vi "VI Server_Test_Slots_TREE_PopulateTreeItems.vi"(4 "Item Names":string[][](array[string])=[["Setting NI-USB6343 digital and analog outputs", "0", "", "", "", "", "", ""], ["Setting digital output and input", "1", "Sets port 0/line 1 to Hi", "Digital input port0/line0 shall be Hi", "", "", "", ""], ["DPO2012B,SET,OS.Ch2.Enbl,ON,", "1", "NI-USB6343,SET,AO.SampleMode,Continious Samples,", "NI-USB6343,SET,AO.MaxVoltage,10.000,", "", "", "", ""], ["DPO2012B: Get the waveform for Graph 2", "1", "Gets the waveform for Graph 2 from DPO2012B.", "", "", "", "", ""], ["Keithley2100,SET,*RST,ON,", "1", "NI-USB6343,SET,AO.Output,OFF,", "NI-USB6343,SET,AO.Physical.Channel,NI-USB6343/ao1,", "", "", "", ""], ["Test EXI-8000PCI MIL-1553 Board", "0", "EXI-8000PCI MIL-1553 Board module 0 shall be set as BC (Buss Controller) and the module 1 shall be set as RT.", "The board shall perform BC2RT, RT2BC and BM (bus monitor) functions.", "", "", "", ""], ["EXI-8000PCIe,SET,RT.Start,OFF,", "2", "EXI-8000PCIe,SET,BC.Mode,BC/CONCURRENT RT,", "EXI-8000PCIe,SET,BC.RT.Number,1,", "", "", "", ""], ["EXI-8000PCIe,SET,RT.Start,OFF,", "2", "EXI-8000PCIe,SET,BC.Mode,BC/CONCURRENT RT,", "EXI-8000PCIe,SET,BC.RT.Number,1,", "", "", "", ""], ["Delay,,,250,", "1", "EXI-8000PCIe,SET,BC.Mode,BC/CONCURRENT RT,", "EXI-8000PCIe,SET,BC.RT.Number,1,", "", "", "", ""], ["EXI-8000PCIe,SET,RT.Start,OFF,", "1", "EXI-8000PCIe,SET,BC.Mode,BC/CONCURRENT RT,", "EXI-8000PCIe,SET,BC.RT.Number,1,", "", "", "", ""], ["Test SRS 5330A and API 8810A", "0", "Testing synchroresolver instruments", "", "", "", "", ""], ["Setting SRS 5330A", "1", "Testing SRS 5330A functions", "Testing SRS 5330A functions", "", "", "", ""], ["API 8810A Functions test", "1", "Perfoms API 8810A Functions test", "", "", "", "", ""], ["Demo test", "1", "Demo Test: create test case", "", "", "", "", ""], ["DPO2012B,SET,OS.Ch2.Enbl,ON,", "1", "NI-USB6343,SET,AO.SampleMode,Continious Samples,", "NI-USB6343,SET,AO.MaxVoltage,10.000,", "", "", "", ""]], 6 "Tree.RowHeaders":string[](array[string]), 7 "Label":string="Test.Tree", 8 "error in":errorcluster, 9 "Tree.Ref":refnum<vi>, 11 "VI Server.RefsCluster":T1={"Labels"=["Tab.Main", "EXIT", "Test.Start", "Test.ABORT", "Test.Pause", "error in", "error out", "Login.Level", "Login.Name", "TestConfiguration.TestCaseEdit", "TestConfiguration.DeleteTestCase", "TestConfiguration.P/N.TestCaseNew", "TestConfiguration.SaveTestCase", "Settings.TestCase.Refresh", "Help", "System.Message", "Instruments.Status", "Test.Tree", "Serial#", "Test.P/N", "Messages & Status", "Settings.P/N", "TestCase", "TestConfiguration", "TestCase.Description", "TestCase.Conditions", "TestCase.Parameter", "TestCaseConfiguration", "TestCase.TraceLimits", "TestCase.Function", "TestCase.Function.Argument1", "TestCase.Function.Argument2", "TestCase.Function.Argument3", "TestCase.Function.Argument3.DBL", "TestCase.LimitsIndex", "LimitsIndex.New", "Limit.Hi", "Limit.Lo", "Limit.Units", "Limits.SAVE", "Limits.Remove", "TestCase.Instrument.Data", "TestCase.InstrumentData.InRange", "TestCase.Execute.Selected", "TestCase.Execute.All", "TestCase.Execute.Pause", "TestCase.Execute.ABORT", "TestCase.Execute.Instruction", "TestCase.Add.Instruction", "TestCase.SAVE", "TestCase.Instrument.Data.Array", "TestCase.Execution.StepTime", "TestCase.Update.Instruction", "Limit.Message", "TestCase.Execute.Pass/Fail", "Performance.Verification.Pass/Fail", "Performance.Verification.SAVE", "TestCase.Execute.Next", "TestConfiguration.RunAll", "TestConfiguration.Execute.Pass/Fail", "TestCaseExecution.StopOnFailure", "TestConfiguration.Run.Step", "TestCase.Add.Instruction.Pos", "TestCase.Execute.Steps", "TestCase.Execute.Step.Pause", "Graph1", "Graph2", "Image1", "Image2", "Image3", "Mem1", "Mem2", "Mem3", "Mem4", "Mem5", "Mem6", "Mem7", "Mem8", "Mem9", "Mem10", "Mem11", "Mem12", "Mem13", "Mem14", "Mem15", "Mem16", "Mem97", "Mem98", "Mem99", "Mem100", "Mem101", "Mem102", "Mem103", "Mem104", "Mem105", "Mem106", "Mem107", "Mem108", "Mem109", "Mem110", "Mem111", "Mem112", "Mem17", "Mem18", "Mem19", "Mem20", "Mem21", "Mem22", "Mem23", "Mem24", "Mem25", "Mem26", "Mem27", "Mem28", "Mem29", "Mem30", "Mem31", "Mem32", "Mem113", "Mem114", "Mem115", "Mem116", "Mem117", "Mem118", "Mem119", "Mem120", "Mem121", "Mem122", "Mem123", "Mem124", "Mem125", "Mem126", "Mem127", "Mem128", "Mem33", "Mem34", "Mem35", "Mem36", "Mem37", "Mem38", "Mem39", "Mem40", "Mem41", "Mem42", "Mem43", "Mem44", "Mem45", "Mem46", "Mem47", "Mem48", "Mem129", "Mem130", "Mem131", "Mem132", "Mem133", "Mem134", "Mem135", "Mem136", "Mem137", "Mem138", "Mem139", "Mem140", "Mem141", "Mem142", "Mem143", "Mem144", "Mem49", "Mem50", "Mem51", "Mem52", "Mem53", "Mem54", "Mem55", "Mem56", "Mem57", "Mem58", "Mem59", "Mem60", "Mem61", "Mem62", "Mem63", "Mem64", "Mem145", "Mem146", "Mem147", "Mem148", "Mem149", "Mem150", "Mem151", "Mem152", "Mem153", "Mem154", "Mem155", "Mem156", "Mem157", "Mem158", "Mem159", "Mem160", "Mem65", "Mem66", "Mem67", "Mem68", "Mem69", "Mem70", "Mem71", "Mem72", "Mem73", "Mem74", "Mem75", "Mem76", "Mem77", "Mem78", "Mem79", "Mem80", "Mem161", "Mem162", "Mem163", "Mem164", "Mem165", "Mem166", "Mem167", "Mem168", "Mem169", "Mem170", "Mem171", "Mem172", "Mem173", "Mem174", "Mem175", "Mem176", "Mem81", "Mem82", "Mem83", "Mem84", "Mem85", "Mem86", "Mem87", "Mem88", "Mem89", "Mem90", "Mem91", "Mem92", "Mem93", "Mem94", "Mem95", "Mem96", "Mem177", "Mem178", "Mem179", "Mem180", "Mem181", "Mem182", "Mem183", "Mem184", "Mem185", "Mem186", "Mem187", "Mem188", "Mem189", "Mem190", "Mem191", "Mem192", "System.SupportedPartNumbers", "System.PartNumber", "System.Instruments", "System.NewInstrument.Name", "System.NewInstrument.Tag", "System.NewInstrument.Path", "UDP.IP.Address", "UDP.LocalPort", "UDP.Port.BC", "UDP.Port.RT", "UDP.Test.String", "UDP.Responce.String", "UDP.Responce.String.Monitor", "UDP.Test.String.Send", "Instr.Responce.Timeout", "UDP.Sent.String", "Performance.Verification.Enable", "UDP.Responce.Array", "UDP.Write.Array", "TestCase.Diagnostics.ABORT", "TestCase.Diagnostics.Pause", "TestCase.Diagnostics.Next", "TestCase.Diagnostics.Instruction", "InstrumentLoad.Disable"], "Refs"=[refnum, refnum, refnum, refnum, refnum, refnum, refnum, refnum, refnum, refnum, refnum, refnum, refnum, refnum, refnum, refnum, refnum, refnum, refnum, refnum, refnum, refnum, refnum, refnum, refnum, refnum, refnum, refnum, refnum, refnum, refnum, refnum, refnum, refnum, refnum, refnum, refnum, refnum, refnum, refnum, refnum, refnum, refnum, refnum, refnum, refnum, refnum, refnum, refnum, refnum, refnum, refnum, refnum, refnum, refnum, refnum, refnum, refnum, refnum, refnum, refnum, refnum, refnum, refnum, refnum, refnum, refnum, refnum, refnum, refnum, refnum, refnum, refnum, refnum, refnum, refnum, refnum, refnum, refnum, refnum, refnum, refnum, refnum, refnum, refnum, refnum, refnum, refnum, refnum, refnum, refnum, refnum, refnum, refnum, refnum, refnum, refnum, refnum, refnum, refnum, refnum, refnum, refnum, refnum, refnum, refnum, refnum, refnum, refnum, refnum, refnum, refnum, refnum, refnum, refnum, refnum, refnum, refnum, refnum, refnum, refnum, refnum, refnum, refnum, refnum, refnum, refnum, refnum, refnum, refnum, refnum, refnum, refnum, refnum, refnum, refnum, refnum, refnum, refnum, refnum, refnum, refnum, refnum, refnum, refnum, refnum, refnum, refnum, refnum, refnum, refnum, refnum, refnum, refnum, refnum, refnum, refnum, refnum, refnum, refnum, refnum, refnum, refnum, refnum, refnum, refnum, refnum, refnum, refnum, refnum, refnum, refnum, refnum, refnum, refnum, refnum, refnum, refnum, refnum, refnum, refnum, refnum, refnum, refnum, refnum, refnum, refnum, refnum, refnum, refnum, refnum, refnum, refnum, refnum, refnum, refnum, refnum, refnum, refnum, refnum, refnum, refnum, refnum, refnum, refnum, refnum, refnum, refnum, refnum, refnum, refnum, refnum, refnum, refnum, refnum, refnum, refnum, refnum, refnum, refnum, refnum, refnum, refnum, refnum, refnum, refnum, refnum, refnum, refnum, refnum, refnum, refnum, refnum, refnum, refnum, refnum, refnum, refnum, refnum, refnum, refnum, refnum, refnum, refnum, refnum, refnum, refnum, refnum, refnum, refnum, refnum, refnum, refnum, refnum, refnum, refnum, refnum, refnum, refnum, refnum, refnum, refnum, refnum, refnum, refnum, refnum, refnum, refnum, refnum, refnum, refnum, refnum, refnum, refnum, refnum, refnum, refnum, refnum, refnum, refnum, refnum, refnum, refnum, refnum, refnum, refnum], "VI Ref"=refnum}) -> (0 "error out":errorcluster={"status"=TRUE, "code"=1088, "source"="Invoke Node in VI Server_TREE_PopulateTreeItems.vi->ExEng_Init_TestTree.vi->ExEng_INIT_Main.vi->ExecutionEngine_MAIN.vi\n<APPEND>\nMethod Name: <b>Edit Tree Items:Add Item to End</b>"}, 1 "Tree.Ref.DUP":refnum<vi>, 3 "VI Server.RefsCluster.DUP":T1={"Labels"=["Tab.Main", "EXIT", "Test.Start", "Test.ABORT", "Test.Pause", "error in", "error out", "Login.Level", "Login.Name", "TestConfiguration.TestCaseEdit", "TestConfiguration.DeleteTestCase", "TestConfiguration.P/N.TestCaseNew", "TestConfiguration.SaveTestCase", "Settings.TestCase.Refresh", "Help", "System.Message", "Instruments.Status", "Test.Tree", "Serial#", "Test.P/N", "Messages & Status", "Settings.P/N", "TestCase", "TestConfiguration", "TestCase.Description", "TestCase.Conditions", "TestCase.Parameter", "TestCaseConfiguration", "TestCase.TraceLimits", "TestCase.Function", "TestCase.Function.Argument1", "TestCase.Function.Argument2", "TestCase.Function.Argument3", "TestCase.Function.Argument3.DBL", "TestCase.LimitsIndex", "LimitsIndex.New", "Limit.Hi", "Limit.Lo", "Limit.Units", "Limits.SAVE", "Limits.Remove", "TestCase.Instrument.Data", "TestCase.InstrumentData.InRange", "TestCase.Execute.Selected", "TestCase.Execute.All", "TestCase.Execute.Pause", "TestCase.Execute.ABORT", "TestCase.Execute.Instruction", "TestCase.Add.Instruction", "TestCase.SAVE", "TestCase.Instrument.Data.Array", "TestCase.Execution.StepTime", "TestCase.Update.Instruction", "Limit.Message", "TestCase.Execute.Pass/Fail", "Performance.Verification.Pass/Fail", "Performance.Verification.SAVE", "TestCase.Execute.Next", "TestConfiguration.RunAll", "TestConfiguration.Execute.Pass/Fail", "TestCaseExecution.StopOnFailure", "TestConfiguration.Run.Step", "TestCase.Add.Instruction.Pos", "TestCase.Execute.Steps", "TestCase.Execute.Step.Pause", "Graph1", "Graph2", "Image1", "Image2", "Image3", "Mem1", "Mem2", "Mem3", "Mem4", "Mem5", "Mem6", "Mem7", "Mem8", "Mem9", "Mem10", "Mem11", "Mem12", "Mem13", "Mem14", "Mem15", "Mem16", "Mem97", "Mem98", "Mem99", "Mem100", "Mem101", "Mem102", "Mem103", "Mem104", "Mem105", "Mem106", "Mem107", "Mem108", "Mem109", "Mem110", "Mem111", "Mem112", "Mem17", "Mem18", "Mem19", "Mem20", "Mem21", "Mem22", "Mem23", "Mem24", "Mem25", "Mem26", "Mem27", "Mem28", "Mem29", "Mem30", "Mem31", "Mem32", "Mem113", "Mem114", "Mem115", "Mem116", "Mem117", "Mem118", "Mem119", "Mem120", "Mem121", "Mem122", "Mem123", "Mem124", "Mem125", "Mem126", "Mem127", "Mem128", "Mem33", "Mem34", "Mem35", "Mem36", "Mem37", "Mem38", "Mem39", "Mem40", "Mem41", "Mem42", "Mem43", "Mem44", "Mem45", "Mem46", "Mem47", "Mem48", "Mem129", "Mem130", "Mem131", "Mem132", "Mem133", "Mem134", "Mem135", "Mem136", "Mem137", "Mem138", "Mem139", "Mem140", "Mem141", "Mem142", "Mem143", "Mem144", "Mem49", "Mem50", "Mem51", "Mem52", "Mem53", "Mem54", "Mem55", "Mem56", "Mem57", "Mem58", "Mem59", "Mem60", "Mem61", "Mem62", "Mem63", "Mem64", "Mem145", "Mem146", "Mem147", "Mem148", "Mem149", "Mem150", "Mem151", "Mem152", "Mem153", "Mem154", "Mem155", "Mem156", "Mem157", "Mem158", "Mem159", "Mem160", "Mem65", "Mem66", "Mem67", "Mem68", "Mem69", "Mem70", "Mem71", "Mem72", "Mem73", "Mem74", "Mem75", "Mem76", "Mem77", "Mem78", "Mem79", "Mem80", "Mem161", "Mem162", "Mem163", "Mem164", "Mem165", "Mem166", "Mem167", "Mem168", "Mem169", "Mem170", "Mem171", "Mem172", "Mem173", "Mem174", "Mem175", "Mem176", "Mem81", "Mem82", "Mem83", "Mem84", "Mem85", "Mem86", "Mem87", "Mem88", "Mem89", "Mem90", "Mem91", "Mem92", "Mem93", "Mem94", "Mem95", "Mem96", "Mem177", "Mem178", "Mem179", "Mem180", "Mem181", "Mem182", "Mem183", "Mem184", "Mem185", "Mem186", "Mem187", "Mem188", "Mem189", "Mem190", "Mem191", "Mem192", "System.SupportedPartNumbers", "System.PartNumber", "System.Instruments", "System.NewInstrument.Name", "System.NewInstrument.Tag", "System.NewInstrument.Path", "UDP.IP.Address", "UDP.LocalPort", "UDP.Port.BC", "UDP.Port.RT", "UDP.Test.String", "UDP.Responce.String", "UDP.Responce.String.Monitor", "UDP.Test.String.Send", "Instr.Responce.Timeout", "UDP.Sent.String", "Performance.Verification.Enable", "UDP.Responce.Array", "UDP.Write.Array", "TestCase.Diagnostics.ABORT", "TestCase.Diagnostics.Pause", "TestCase.Diagnostics.Next", "TestCase.Diagnostics.Instruction", "InstrumentLoad.Disable"], "Refs"=[refnum, refnum, refnum, refnum, refnum, refnum, refnum, refnum, refnum, refnum, refnum, refnum, refnum, refnum, refnum, refnum, refnum, refnum, refnum, refnum, refnum, refnum, refnum, refnum, refnum, refnum, refnum, refnum, refnum, refnum, refnum, refnum, refnum, refnum, refnum, refnum, refnum, refnum, refnum, refnum, refnum, refnum, refnum, refnum, refnum, refnum, refnum, refnum, refnum, refnum, refnum, refnum, refnum, refnum, refnum, refnum, refnum, refnum, refnum, refnum, refnum, refnum, refnum, refnum, refnum, refnum, refnum, refnum, refnum, refnum, refnum, refnum, refnum, refnum, refnum, refnum, refnum, refnum, refnum, refnum, refnum, refnum, refnum, refnum, refnum, refnum, refnum, refnum, refnum, refnum, refnum, refnum, refnum, refnum, refnum, refnum, refnum, refnum, refnum, refnum, refnum, refnum, refnum, refnum, refnum, refnum, refnum, refnum, refnum, refnum, refnum, refnum, refnum, refnum, refnum, refnum, refnum, refnum, refnum, refnum, refnum, refnum, refnum, refnum, refnum, refnum, refnum, refnum, refnum, refnum, refnum, refnum, refnum, refnum, refnum, refnum, refnum, refnum, refnum, refnum, refnum, refnum, refnum, refnum, refnum, refnum, refnum, refnum, refnum, refnum, refnum, refnum, refnum, refnum, refnum, refnum, refnum, refnum, refnum, refnum, refnum, refnum, refnum, refnum, refnum, refnum, refnum, refnum, refnum, refnum, refnum, refnum, refnum, refnum, refnum, refnum, refnum, refnum, refnum, refnum, refnum, refnum, refnum, refnum, refnum, refnum, refnum, refnum, refnum, refnum, refnum, refnum, refnum, refnum, refnum, refnum, refnum, refnum, refnum, refnum, refnum, refnum, refnum, refnum, refnum, refnum, refnum, refnum, refnum, refnum, refnum, refnum, refnum, refnum, refnum, refnum, refnum, refnum, refnum, refnum, refnum, refnum, refnum, refnum, refnum, refnum, refnum, refnum, refnum, refnum, refnum, refnum, refnum, refnum, refnum, refnum, refnum, refnum, refnum, refnum, refnum, refnum, refnum, refnum, refnum, refnum, refnum, refnum, refnum, refnum, refnum, refnum, refnum, refnum, refnum, refnum, refnum, refnum, refnum, refnum, refnum, refnum, refnum, refnum, refnum, refnum, refnum, refnum, refnum, refnum, refnum, refnum, refnum, refnum, refnum, refnum, refnum, refnum, refnum, refnum, refnum, refnum, refnum, refnum, refnum, refnum], "VI Ref"=refnum})   [LabVIEW 2020]
uses:
  VI Server_TypeDefs/VI Server_RefsCluster.ctl
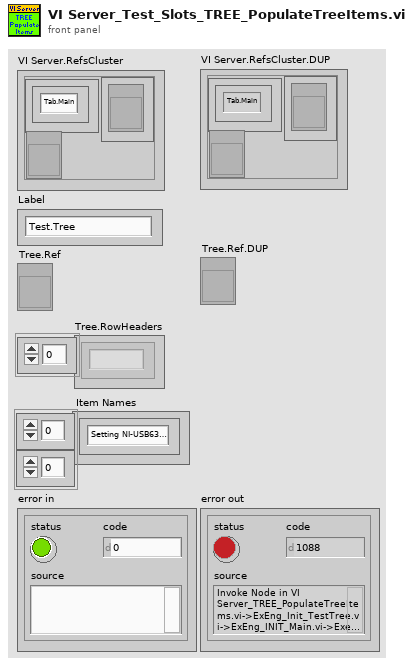
[diagram p1: front panel]
types:
  T1 = typedef "VI Server_RefsCluster.ctl" = cluster{"Labels":string[], "Refs":refnum<vi>[], "VI Ref":refnum<vi>}
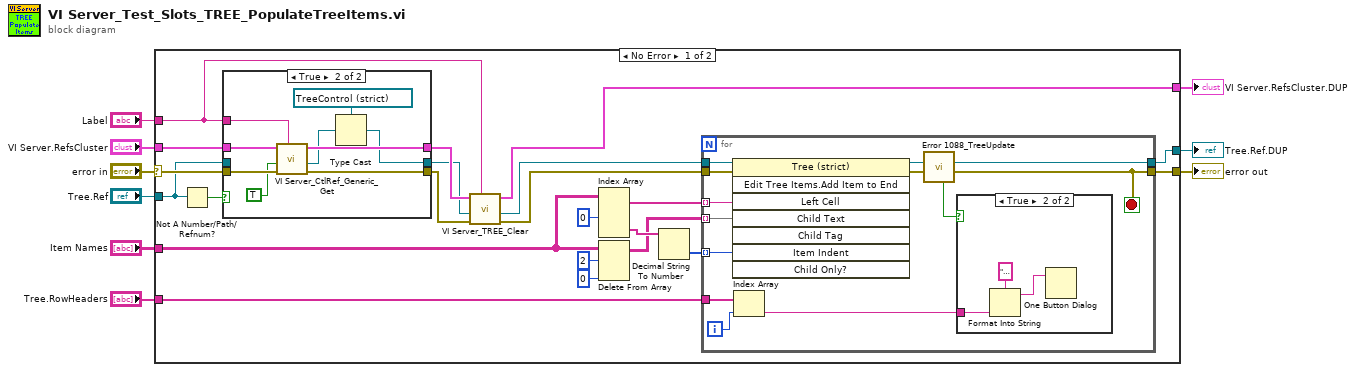
[diagram p0: block diagram]
diagram:
  n1 = case shown="No Error" "error in" {
    selector: "error in" -> [w31 w60]
    tunnel: [w20 w60] -> w8
    tunnel: "VI Server.RefsCluster" -> [w30 w59]
    tunnel: [w15 w59] -> w1
    tunnel: "Label" -> [w12 _]
    tunnel: [w19 _] -> w4
    tunnel: "Tree.Ref" -> [w28 _]
    tunnel: "Item Names" -> [w18 _]
    tunnel: "Tree.RowHeaders" -> [w17 _]
    frame No Error {
      n2 = Not A Number/Path/Refnum?(number/path/refnum=w28) -> (NaN/Path/Refnum?=w29:bool)
      n3 = case shown="True" w29 {
        tunnel: w31 -> [w49 w58]
        tunnel: w30 -> [w48 w57]
        tunnel: [w48 w56] -> w16
        tunnel: w12 -> [_ w55]
        tunnel: [w49 w53] -> w14
        tunnel: w28 -> [w47 _]
        tunnel: [w47 w52] -> w11
        frame False {
        }
        frame True {
          n4 = call "VI Server_CtlRef_Generic_Get.vi"("Control.Label"=w55, "error in"=w58, "SingleInstance"=TRUE, "VI Server.RefsCluster"=w57) -> ("error out"=w53:errorcluster, "Control.Ref.Generic"=w54:refnum<vi>, "VI Server.RefsCluster.DUP"=w56:T1)  [unwired: 5 in]
          n5 = Type Cast(type=refnum<vi> refnum ("Test.Tree"), x=w54) -> (*(type *) &x=w52:refnum<vi>)
        }
      }
      n6 = call "VI Server_TREE_Clear.vi"("Label"=w12, "error in"=w14, "Tree.Ref"=w11, "VI Server.RefsCluster"=w16) -> ("error out"=w13:errorcluster, "Tree.Ref.DUP"=w10:refnum<vi>, "VI Server.RefsCluster.DUP"=w15:T1)  [unwired: 5 in]
      n7 = Index Array(array=w18, index (col) #1=0 ("disabled index (col)")) -> (element #1=w26:string[], element #2=w25:string[])  [unwired: 3 in]
      n8 = Delete From Array(array=w18, length=2, index (col)=0 ("disabled index (col)")) -> (array with subset deleted=w21:string[][])  [unwired: 1 in, 1 out]
      n9 = Decimal String To Number(string=w25) -> (number=w24:i32[])  [unwired: 2 in, 1 out]
      n10 = for {
        tunnel: w26 -> [w42] mode=indexing
        tunnel: w24 -> [w41] mode=indexing
        tunnel: w21 -> [w40] mode=indexing
        tunnel: [w39] -> w19
        tunnel: w13 -> [w43]
        tunnel: [w34] -> w20
        tunnel: w10 -> [w38]
        tunnel: w17 -> [w36]
        i -> [w37]
        stop <- w34 stop-if-true
        # "Populate the tree items"
        n11 = invoke on="Invoke Node" class="Tree (strict)" method="Edit Tree Items.Add Item to End"(reference=w38, error in=w43, "Left Cell"=w42, "Child Text"=w40, "Item Indent"=w41) -> (reference out=w39:refnum<vi>, error out=w35:errorcluster)  [unwired: 3 in, 6 out]
        n12 = Index Array(array=w36, index=w37) -> (element=w32:string)
        n13 = call "Error 1088_TreeUpdate.vi"("error in"=w35) -> ("error out"=w34:errorcluster, "Error.1088"=w33:bool)  [unwired: 9 in]
        n14 = case shown="True" w33 {
          tunnel: w32 -> [_ w46]
          frame False {
          }
          frame True {
            n15 = Format Into String(format string="Error loading Teast Case #%s.\nPossible Reason:\nThere is no parent item for this test case.\nAs an example, if the test case number is 2.1.1, there MUST be\nthe test case/item with number of 2.1", w46) -> (resulting string=w44:string)  [unwired: 2 in, 1 out]
            n16 = One Button Dialog(message=w44) -> ()  [unwired: 1 in, 1 out]
          }
        }
      }
    }
    frame Error {
    }
  }
  "VI Server.RefsCluster.DUP" <- w1
  "error out" <- w8
  "Tree.Ref.DUP" <- w4
